vi "Test - Property required.vi"   [LabVIEW 2020, in "JSON Schema Generator.lvlib"]
uses:
  JSON Schema Generator.lvlib
  <vilib>/addons/_JKI Toolkits/Caraya/classes/Test/Test.lvclass
  <vilib>/addons/_JKI Toolkits/Caraya/classes/Assert/Assert.lvclass
  <vilib>/addons/_JKI Toolkits/Caraya/classes/Assert/Assert Equal Value_Variant.vi
  <vilib>/addons/_JKI Toolkits/Caraya/classes/Assert/Assert Not Error.vi
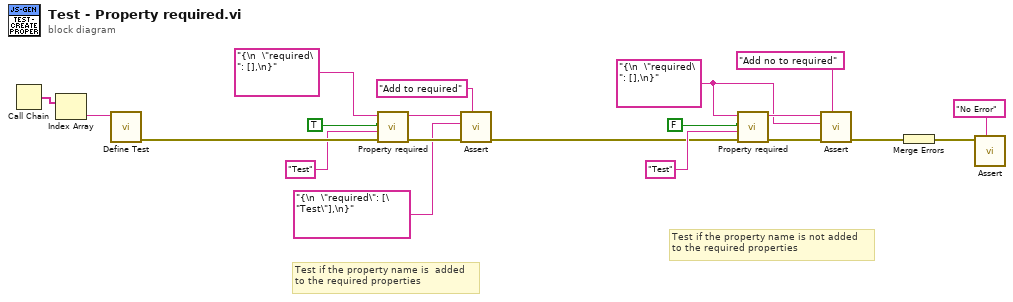
[diagram p0: block diagram]
diagram:
  w2 = "{\n  \"required\": [],\n}" ("JSON Schema in")
  # "Test if the property name is  added\nto the required properties"
  # "Test if the property name is not added\nto the required properties"
  n1 = Call Chain() -> (call chain=w20:string[])
  n2 = Index Array(array=w20) -> (element=w19:string)  [unwired: 1 in]
  n3 = call <vilib>:"Define Test.vi"("Label (VI Title)"=w19) -> ("error out"=w15:errorcluster)  [unwired: 9 in, 1 out]
  n4 = call "Property required.vi"("error in (no error)"=w15, "Name"="Test", "Required?"=TRUE, "JSON Schema in"="{\n  \"required\": [],\n}") -> ("error out"=w14:errorcluster, "JSON Schema out"=w10:string)  [unwired: 6 in]
  n5 = call-poly <vilib>:"Assert.vi"("Label"="Add to required", "error in (no error)"=w14, "Actual"="{\n  \"required\": [\"Test\"],\n}" ("JSON Schema in"), "Expected"=w10) -> ("error out"=w3:errorcluster)  [unwired: 6 in, 1 out]
  n6 = call "Property required.vi"("error in (no error)"=w3, "Name"="Test", "Required?"=FALSE, "JSON Schema in"=w2) -> ("error out"=w5:errorcluster, "JSON Schema out"=w8:string)  [unwired: 6 in]
  n7 = call-poly <vilib>:"Assert.vi"("Label"="Add no to required", "error in (no error)"=w5, "Actual"=w2, "Expected"=w8) -> ("error out"=w1:errorcluster)  [unwired: 6 in, 1 out]
  n8 = Merge Errors(w1) -> (w16:errorcluster)
  n9 = call-poly <vilib>:"Assert.vi"("Label"="No Error", "Not Error?"=w16) -> ()  [unwired: 8 in, 2 out]
